vi "RAwr.vi"() -> ()   [LabVIEW 2009]
panel:
  out "Array":u8[](array[numeric])
  out "Hex":string
  in  "String":string
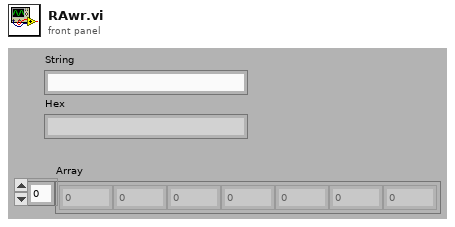
[diagram p1: front panel]
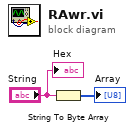
[diagram p0: block diagram]
diagram:
  n1 = String To Byte Array(string="String") -> (unsigned byte array=→"Array":u8[])
  "Hex" <- "String"
